vi "SetupDefault.vi"(8 "error in (no error)":errorcluster, 10 "Alias":string, 11 "PSU_N87 in":refnum<class "PSU_N87.lvclass">) -> (0 "error out":errorcluster, 3 "PSU_N87 out":refnum<class "PSU_N87.lvclass">)   [LabVIEW 2014, in "PSU_N87.lvclass"]
uses:
  PSU_N87.lvclass
  PSU_N87.lvclass/PSU_N87.ctl
  data/Agilent N87XX Series.lvlib
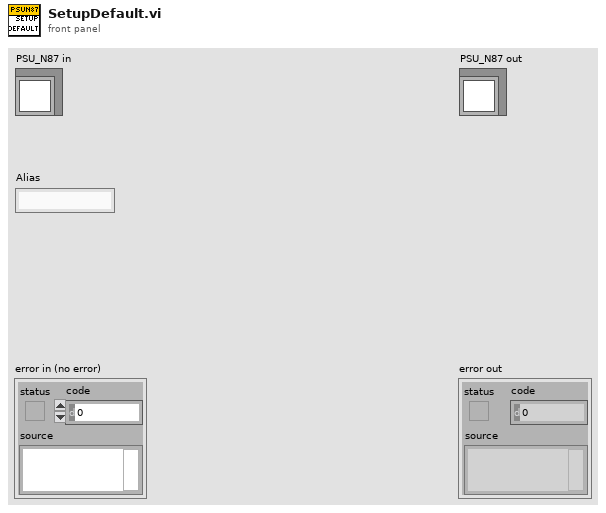
[diagram p1: front panel]
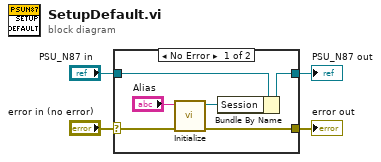
[diagram p0: block diagram]
diagram:
  n1 = case shown="No Error" "error in (no error)" {
    selector: "error in (no error)" -> [w9 w11]
    tunnel: "PSU_N87 in" -> [w7 w12]
    tunnel: [w5 w12] -> w2
    tunnel: [w8 w11] -> w1
    frame No Error {
      n2 = call "Initialize.vi"("error in (no error)"=w9, "VISA resource name"="Alias") -> ("error out"=w8:errorcluster, "VISA resource name out"=w6:refnum<visa-resource-name>)  [unwired: 8 in]
      n3 = Bundle By Name(cluster=w7, "Session"=w6) -> (w5:refnum<class "PSU_N87.lvclass">)
    }
    frame Error {
    }
  }
  "error out" <- w1
  "PSU_N87 out" <- w2
